vi "Read orientation.vi"(8 "error in (no error)":errorcluster, 11 "Robot in":refnum<class "Robot.lvclass">) -> (0 "error out":errorcluster, 2 "orientation":dbl, 3 "Robot out":refnum<class "Robot.lvclass">)   [LabVIEW 2018, in "Robot.lvclass"]
uses:
  Robot.lvclass
  Robot.lvclass/Robot.ctl
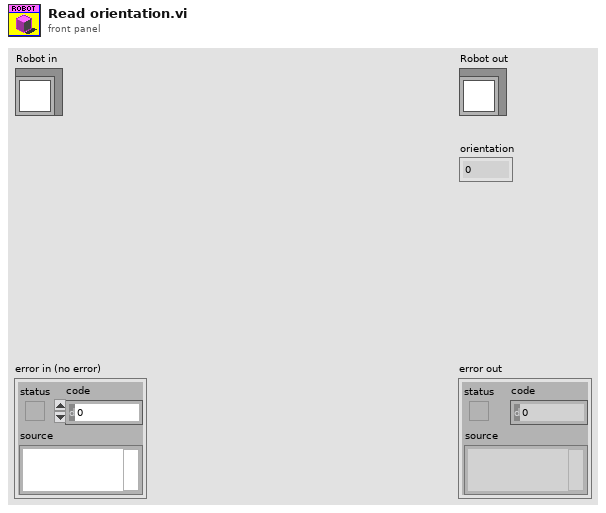
[diagram p1: front panel]
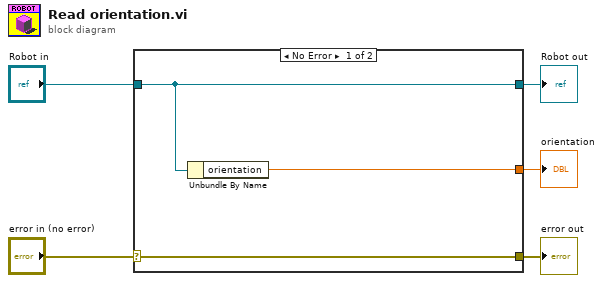
[diagram p0: block diagram]
diagram:
  n1 = case shown="No Error" "error in (no error)" {
    selector: "error in (no error)" -> [w8 w9]
    tunnel: [w8 w9] -> w4
    tunnel: [w7 w10] -> w2
    tunnel: "Robot in" -> [w7 w10]
    tunnel: [w6 _] -> w1
    frame No Error {
      n2 = Unbundle By Name(w7) -> ("orientation"=w6:dbl)
    }
    frame Error {
    }
  }
  "error out" <- w4
  "Robot out" <- w2
  "orientation" <- w1
